vi "Build FilePath By Rule.vi"(8 "error in (no error)":errorcluster, 9 "Time(Empty to Use Current Time)":timestamp, 10 "FileNameRule":T1={"Rule"=enum."TimeBased File Name", "Path"=path "D:/", "filename"="data-%<%m/%d/%Y %H:%M:%S>T.tdms"}) -> (0 "error out":errorcluster, 3 "File":path)   [LabVIEW 2017]
doc: "Builds a file path from FileNameRule, which selects a fixed name, an indexed name or a time-based name. Relative paths are resolved against the application directory, missing folders are created, and the Time input defaults to the current time."
uses:
  _FileName Rule.ctl
  7279ca2d-29ef-4966-b9af-d663423eebb9.vi
  Path Type -- Enum.vi
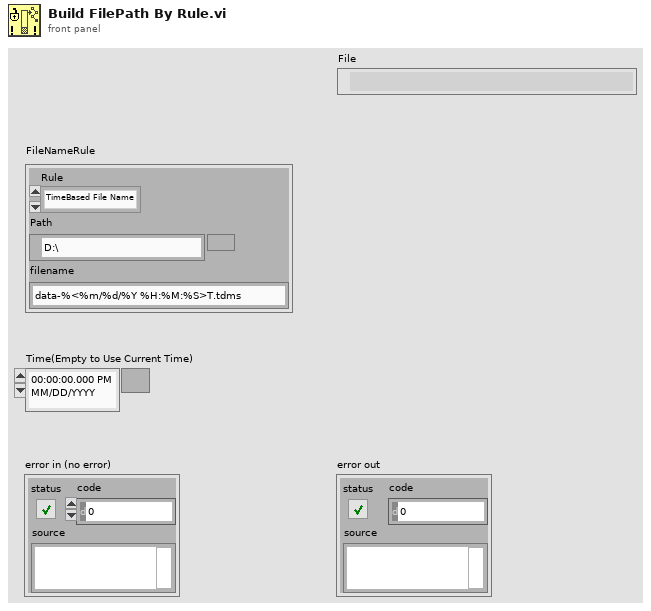
[diagram p1: front panel]
types:
  T1 = typedef "_FileName Rule.ctl" = cluster{"Rule":enum16{"Fixed File Name", "Indexed File Name", "TimeBased File Name"}, "Path":path, "filename":string}
  T2 = enum16{"Fixed File Name", "Indexed File Name", "TimeBased File Name"}
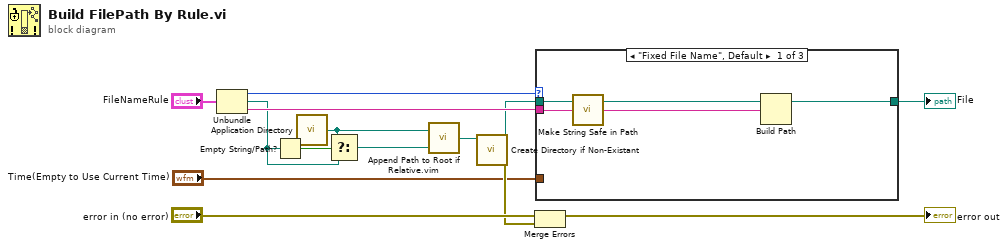
[diagram p0: block diagram]
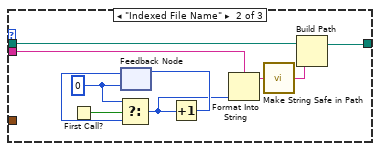
[diagram p2: hidden frame]
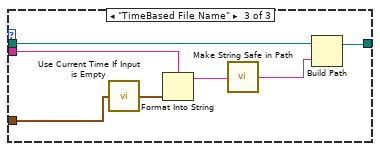
[diagram p3: hidden frame]
diagram:
  n1 = Unbundle("FileNameRule") -> ("Rule"=w14:T2, "Path"=w9:path, "filename"=w13:string)
  n2 = Empty String/Path?(string/path=w9) -> (empty?=w10:bool)
  n3 = call <vilib>:"Application Directory.vi"() -> ("Application Directory"=w4:path)
  n4 = Select(t=w4, s=w10, f=w9) -> (s? t:f=w3:path)
  n5 = call "Append Path to Root if Relative.vim"("Absolute or Relative Path(Scale or Array)"=w3, "Root Path"=w4) -> ("Absolute or Appended Path"=w2:path)
  n6 = call "Create Directory if Non-Existant.vi"("Directory Path"=w2) -> ("error out"=w5:errorcluster, "dup Directory Path"=w12:path)  [unwired: 8 in, 1 out]
  n7 = Merge Errors("error in (no error)", w5) -> (→"error out":errorcluster)
  n8 = case shown="\"Fixed File Name\", Default" w14 {
    tunnel: w12 -> [w18 w26 w34]
    tunnel: w13 -> [w17 w28 w35]
    tunnel: [w16 w25 w33] -> w8
    tunnel: "Time(Empty to Use Current Time)" -> [_ _ w29]
    frame "Fixed File Name", Default {
      n9 = call "Make String Safe in Path.vi"("String In"=w17) -> ("Filesafe String Out"=w15:string)  [unwired: 6 in]
      n10 = Build Path(base path=w18, name or relative path=w15) -> (appended path=w16:path)
    }
    frame "Indexed File Name" {
      w20 = 0 ("t")
      n11 = First Call?() -> (First Call?: T/F=w23:bool)
      n12 = feedback #1(w20) -> (w22:i32)
      n13 = Select(t=w20, s=w23, f=w22) -> (s? t:f=w19:i32)
      n14 = Increment(x=w19) -> (x+1=w21:i32)
      n15 = feedback-in #1(w21) -> ()
      n16 = Format Into String(format string=w28, w19) -> (resulting string=w27:string)  [unwired: 2 in, 1 out]
      n17 = call "Make String Safe in Path.vi"("String In"=w27) -> ("Filesafe String Out"=w24:string)  [unwired: 6 in]
      n18 = Build Path(base path=w26, name or relative path=w24) -> (appended path=w25:path)
    }
    frame "TimeBased File Name" {
      n19 = call "Use Current Time If Input is Empty.vi"("Time(Empty to Use Current Time)"=w29) -> ("Time out"=w30:timestamp)
      n20 = Format Into String(format string=w35, w30) -> (resulting string=w32:string)  [unwired: 2 in, 1 out]
      n21 = call "Make String Safe in Path.vi"("String In"=w32) -> ("Filesafe String Out"=w31:string)  [unwired: 6 in]
      n22 = Build Path(base path=w34, name or relative path=w31) -> (appended path=w33:path)
    }
  }
  "File" <- w8
